vi "device init.vi"(3 "Enum":enum16{"none", "open", "close"}(ring), 4 "test table":refnum<vi>, 5 "device table":refnum<vi>) -> (0 "error IO":errorcluster, 2 "Cluster":T1)   [LabVIEW 2026]
uses:
  a8c8eb06-0f0b-4a7b-a4b2-85656187fa5a.vi
  <vilib>/Instr/_visa.llb/VISA Configure Serial Port (Instr).vi
panel:
  out "Item Names 2":string[][](array[string])
  out "Item Names":string[][](array[string])
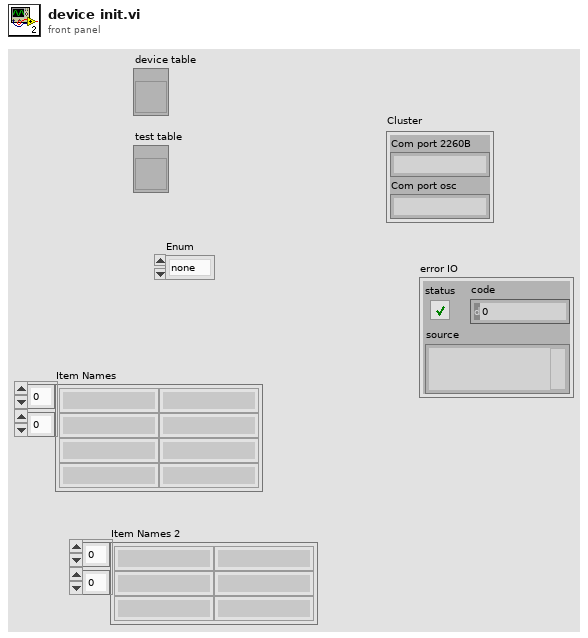
[diagram p1: front panel]
types:
  T1 = cluster{"Com port 2260B":string, "Com port osc":string}
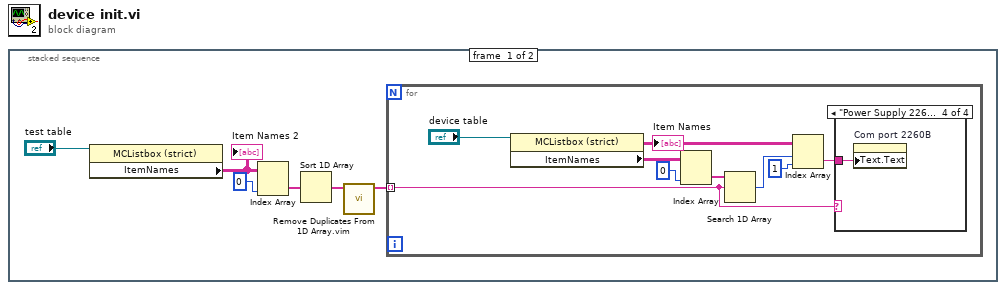
[diagram p0: block diagram]
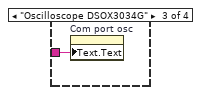
[diagram p4: hidden frame]
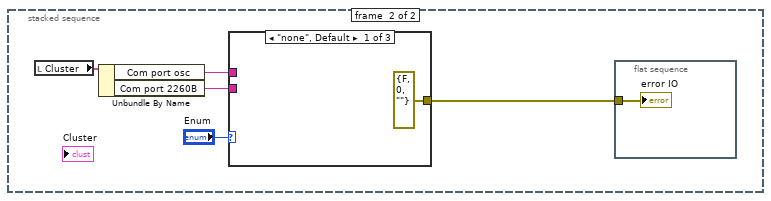
[diagram p5: hidden frame]
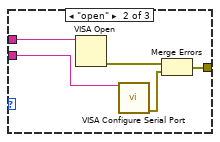
[diagram p6: hidden frame]
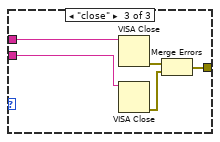
[diagram p7: hidden frame]
diagram:
  n1 = stacked-sequence {
    frame #0 {
      n2 = property class="MCListbox (strict)"(reference="test table") -> ("ItemNames"=w2:string[][])  [unwired: 1 in, 2 out]
      "Item Names 2" <- w2
      n3 = Index Array(array=w2, index (col)=0 ("index (row)")) -> (element=w4:string[])  [unwired: 1 in]
      n4 = Sort 1D Array(array=w4) -> (sorted array=w5:string[])
      n5 = call "Remove Duplicates From 1D Array.vim"("array"=w5) -> ("array with duplicates removed"=w3:string[])  [unwired: 10 in]
      n6 = for {
        tunnel: w3 -> [w10] mode=indexing
        n7 = property class="MCListbox (strict)"(reference="device table") -> ("ItemNames"=w7:string[][])  [unwired: 1 in, 2 out]
        "Item Names" <- w7
        n8 = Index Array(array=w7, index (col)=0 ("index (row)")) -> (element=w13:string[])  [unwired: 1 in]
        n9 = Search 1D Array(1D array=w13, element=w10) -> (index of element=w11:i32)  [unwired: 1 in]
        n10 = Index Array(array=w7, index (row)=w11, index (col)=1 ("disabled index (row)")) -> (element=w9:string)
        n11 = case shown="\"Power Supply 2260B\"" w10 {
          tunnel: w9 -> [_ _ w15 w16]
          frame "False", Default {
          }
          frame "True" {
          }
          frame "Oscilloscope DSOX3034G" {
            n12 = property on="Com port osc" class="Str"("Text.Text"=w15) -> ()  [unwired: 2 in, 2 out]
          }
          frame "Power Supply 2260B" {
            n13 = property on="Com port 2260B" class="Str"("Text.Text"=w16) -> ()  [unwired: 2 in, 2 out]
          }
        }
      }
    }
    frame #1 {
      n14 = local read "Cluster"() -> (w18:T1)
      n15 = Unbundle By Name(w18) -> ("Com port osc"=w20:string, "Com port 2260B"=w21:string)
      n16 = case shown="\"none\", Default" "Enum" {
        tunnel: w20 -> [_ w28 w33]
        tunnel: w21 -> [_ w27 w32]
        tunnel: [errorcluster {"status"=FALSE, "code"=0, "source"=""} ("error IO") w24 w29] -> w17
        frame "none", Default {
        }
        frame "open" {
          n17 = VISA Open(VISA resource name=w28) -> (error out=w26:errorcluster)  [unwired: 4 in, 1 out]
          n18 = call-poly "VISA Configure Serial Port"("VISA resource name"=w27) -> ("error out"=w25:errorcluster)  [unwired: 13 in, 1 out]
          n19 = Merge Errors(w26, w25) -> (w24:errorcluster)
        }
        frame "close" {
          n20 = VISA Close(VISA resource name=w33) -> (error out=w31:errorcluster)  [unwired: 1 in]
          n21 = VISA Close(VISA resource name=w32) -> (error out=w30:errorcluster)  [unwired: 1 in]
          n22 = Merge Errors(w31, w30) -> (w29:errorcluster)
        }
      }
      n23 = flat-sequence {
        tunnel: w17 -> [w22]
        frame #0 {
          "error IO" <- w22
        }
      }
    }
  }
